vi "Addition of sine waves.vi"() -> ()   [LabVIEW 2019]
panel:
  out "Resulting Waveform Chart":dynamicdata(graph)
  out "Waveform Chart 2":dynamicdata(graph)
  in  "Phase 2":dbl caption="Phase"
  in  "Amplitude 2":dbl=1.0 caption="Amplitude"
  in  "Frequency 2":dbl=10.1 caption="Frequency"
  in  "stop":bool
  out "Waveform Chart 1":dynamicdata(graph)
  in  "Phase":dbl
  in  "Amplitude":dbl=1.0
  in  "Frequency":dbl=10.1
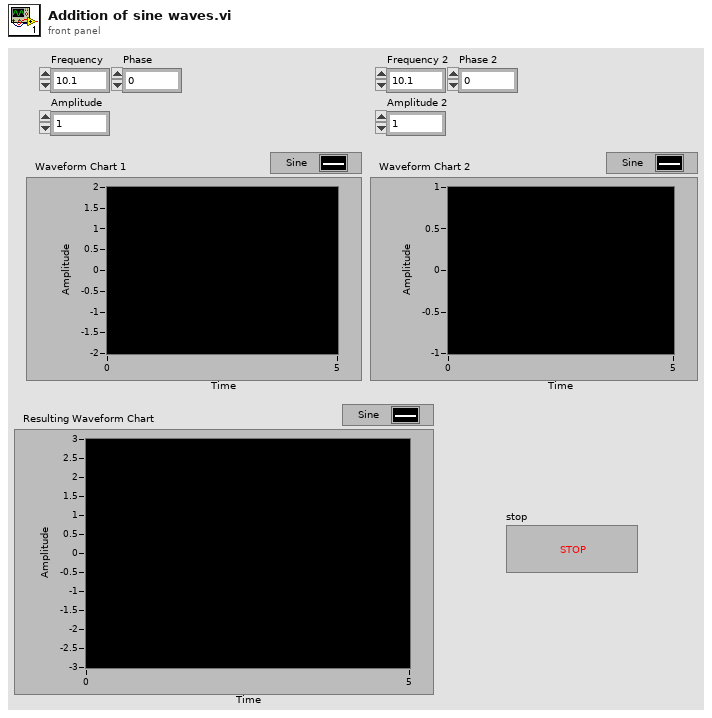
[diagram p1: front panel]
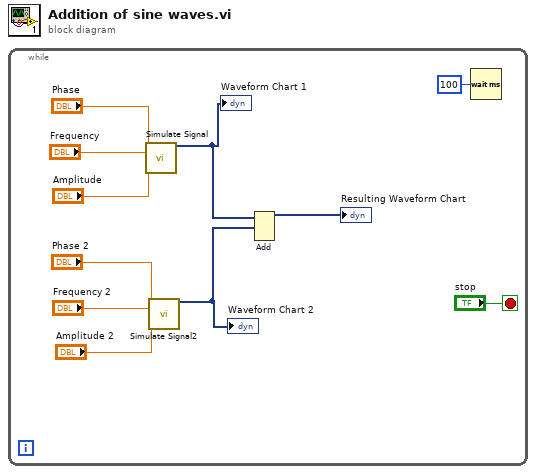
[diagram p0: block diagram]
diagram:
  n1 = while {
    stop <- "stop" stop-if-true
    n2 = call "Simulate Signal"("Frequency"="Frequency", "Amplitude"="Amplitude", "Phase"="Phase") -> ("Sine"=w1:dynamicdata)  [unwired: 11 in, 1 out]
    "Waveform Chart 1" <- w1
    n3 = call "Simulate Signal2"("Frequency"="Frequency 2", "Amplitude"="Amplitude 2", "Phase"="Phase 2") -> ("Sine"=w3:dynamicdata)  [unwired: 11 in, 1 out]
    "Waveform Chart 2" <- w3
    n4 = Add(1:w3, 2:w1) -> (0:→"Resulting Waveform Chart":dynamicdata)  [unwired: 1 in, 1 out]
    n5 = Wait (ms)(milliseconds to wait=u32 100) -> ()  [unwired: 1 out]
  }
